vi "Pass-Fail-Sim.vi"() -> (3 "Boolean":bool)   [LabVIEW 2022 SP3]
panel:
  in  "Fail":bool
  in  "Pass":bool
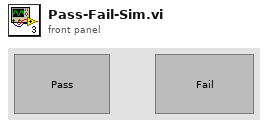
[diagram p1: front panel]
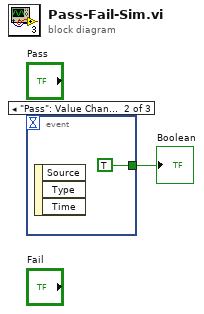
[diagram p0: block diagram]
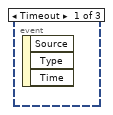
[diagram p2: hidden frame]
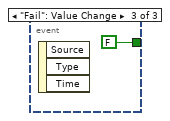
[diagram p3: hidden frame]
diagram:
  n1 = event shown="[1] \"Pass\": Value Change" {
    selector: _ -> [_ _ _]
    dyn-events: _ -> [_ _ _]
    timeout: _ -> [_ _ _]
    tunnel: [_ TRUE FALSE] -> w1
    event Timeout {
      n2 = event-data() -> ()  [unwired: 1 in, 3 out]
    }
    event "Pass": Value Change {
      n3 = event-data() -> ()  [unwired: 1 in, 3 out]
    }
    event "Fail": Value Change {
      n4 = event-data() -> ()  [unwired: 1 in, 3 out]
    }
  }
  "Boolean" <- w1
